vi "Configure Maximum File Count.vi"(8 "Error In":errorcluster, 11 "Maximum":i32) -> (0 "Error Out":errorcluster)   [LabVIEW 2015, in "Logger.lvlib"]
doc: "Sets the maximum number of log files to keep on disk."
uses:
  Logger.lvlib
  Private/File/Action.ctl
  Private/File/File.lvlib
panel:
  # "Zero (0) indicates no pruning, or deleting of old log files."
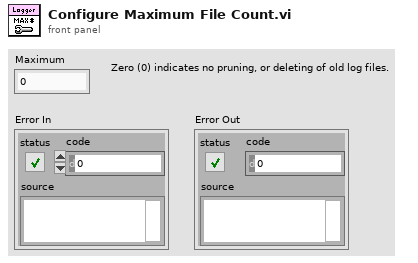
[diagram p1: front panel]
types:
  T1 = typedef "Logger.lvlib/File.lvlib/Action.ctl" = enum16{"Initialize", "Set Maximum File Size", "Set Maximum File Count", "Set Root Folder", "Set Enable Calendar Folder Tree", "Set File Extension", "Start", "Write", "Stop", "Shutdown"}
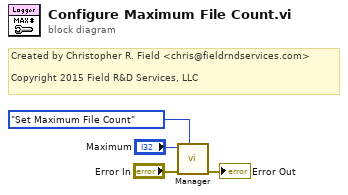
[diagram p0: block diagram]
diagram:
  # "Created by Christopher R. Field <chris@fieldrndservices.com>\n\nCopyright 2015 Field R&D Services, LLC"
  n1 = call "Manager.vi"("Action"=Action."Set Maximum File Count", "Error In"="Error In", "Set Value"="Maximum") -> ("Error Out"=→"Error Out":errorcluster)  [unwired: 8 in]
